vi "convertPercentageToFCVVoltage.vi"(8 "error in (no error)":errorcluster, 10 "Percentage":dbl, 11 "SingleCylinderActuator in":refnum<class "SingleCylinderActuator.lvclass">) -> (0 "error out":errorcluster, 2 "Voltage":dbl, 3 "SingleCylinderActuator out":refnum<class "SingleCylinderActuator.lvclass">)   [LabVIEW 2015, in "SingleCylinderActuator.lvclass"]
uses:
  SingleCylinderActuator.lvclass
  SingleCylinderActuator.lvclass/SingleCylinderActuator.ctl
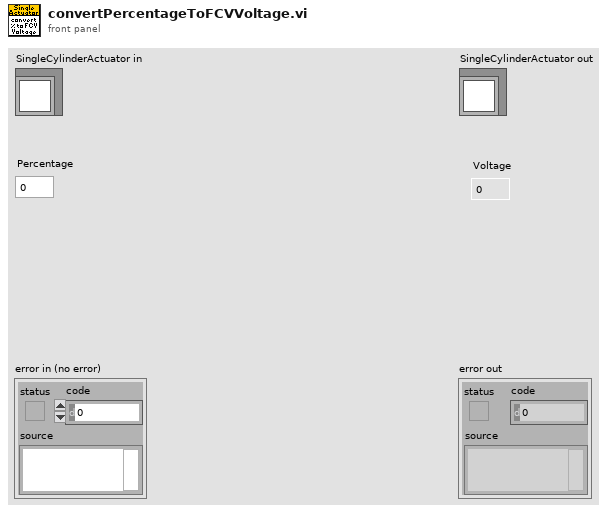
[diagram p1: front panel]
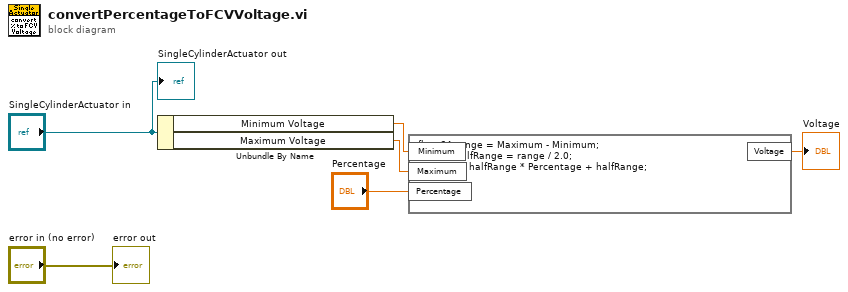
[diagram p0: block diagram]
diagram:
  n1 = Unbundle By Name("SingleCylinderActuator in") -> ("Minimum Voltage"=w2:dbl, "Maximum Voltage"=w1:dbl)
  n2 = formula code="float64 range = Maximum - Minimum;\nfloat64 halfRange = range / 2.0;\nVoltage = halfRange * Percentage + halfRange;"("Minimum"=w2, "Maximum"=w1, "Percentage"="Percentage") -> ("Voltage"=→"Voltage":dbl)
  "error out" <- "error in (no error)"
  "SingleCylinderActuator out" <- "SingleCylinderActuator in"
